vi "Write Configuration File.vi"() -> ()   [LabVIEW 2016]
uses:
  Hardware Configuration Controls/Company.ctl
  Hardware Configuration Controls/Device Type.ctl
  Hardware Configuration Controls/Device Function.ctl
panel:
  in  "Quit":bool
  in  "Save File":bool
  in  "Load File":bool
  in  "Configuration Name":string
  in  "Hardware Configuration Information":T4(array[cluster])
  # "Make sure the 0 element of the array is\nwhere you start putting port/id info"
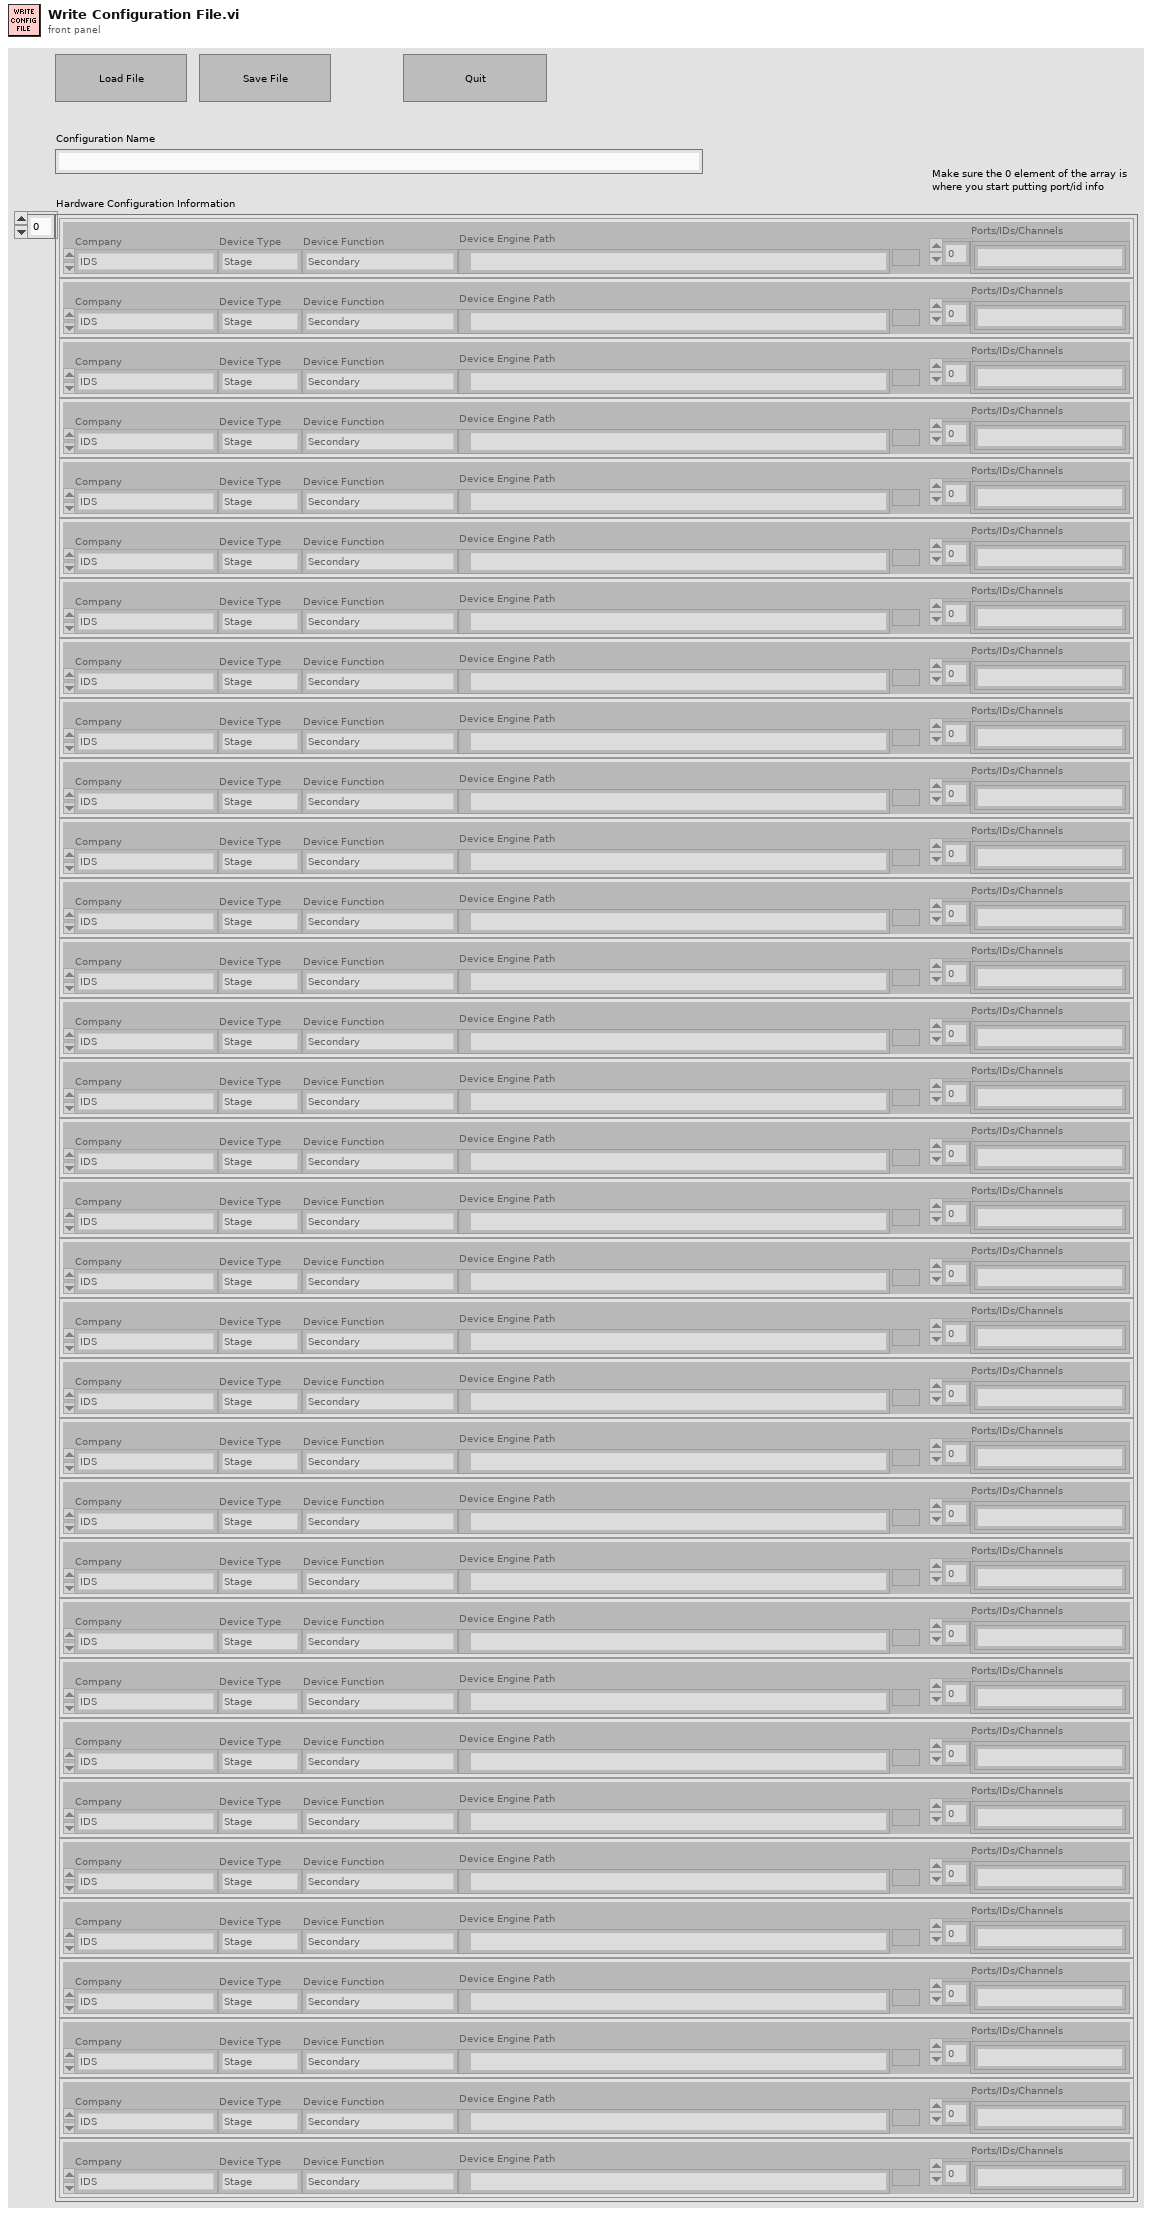
[diagram p1: front panel]
types:
  T1 = typedef "Company.ctl" = enum16{"ASI", "Coherent", "CVI", "Hamamatsu", "IDS", "Mad City Labs", "Marzhauser", "Measurement Computing", "MPB Com", "Photometrics", "PI", "Prior", "Thorlabs"}
  T2 = typedef "Device Type.ctl" = enum16{"AOTF", "Camera", "Deformable Mirror", "Laser", "Shutter", "Stage"}
  T3 = typedef "Device Function.ctl" = enum16{"Primary", "Secondary", "Overview", "Wide Field Drift Correction", "642 nm Excitation", "560 nm Excitation", "546 nm Excitation", "488 nm Excitation", "405 nm Excitation", "Objective Drift Correction", "Objective XY", "Objective Z", "Sample XY", "Sample Coarse Z", "Sample Z", "4Pi Lower", "4Pi Upper", "Adj Cavity"}
  T4 = cluster{"Company":T1, "Device Type":T2, "Device Function":T3, "Device Engine Path":path, "Ports/IDs/Channels":string[]}[]
  T5 = cluster{"Company":T1, "Device Type":T2, "Device Function":T3, path, "Device Port/ID/Channel Info":string[]}
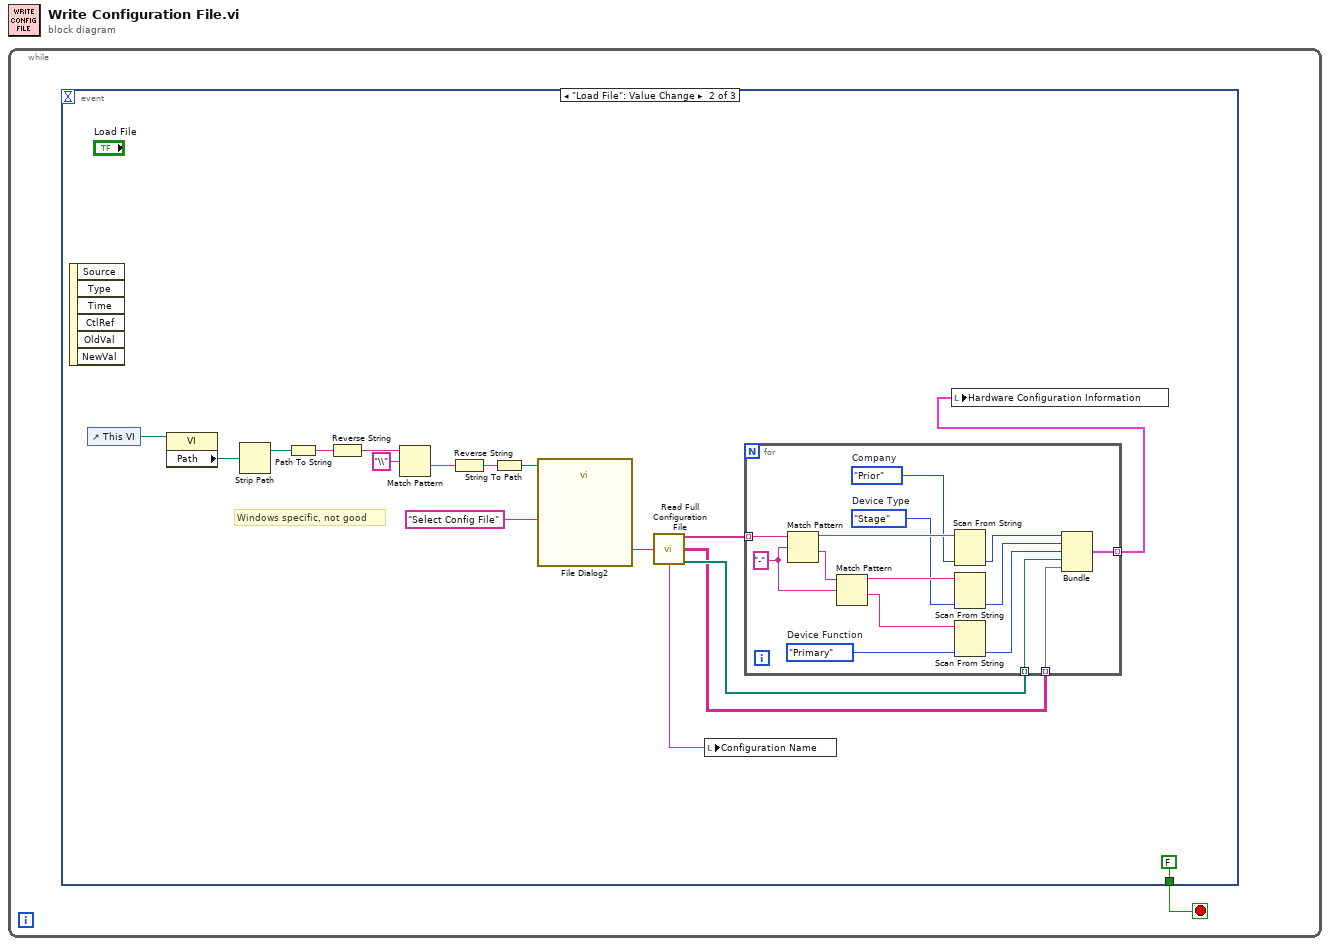
[diagram p0: block diagram]
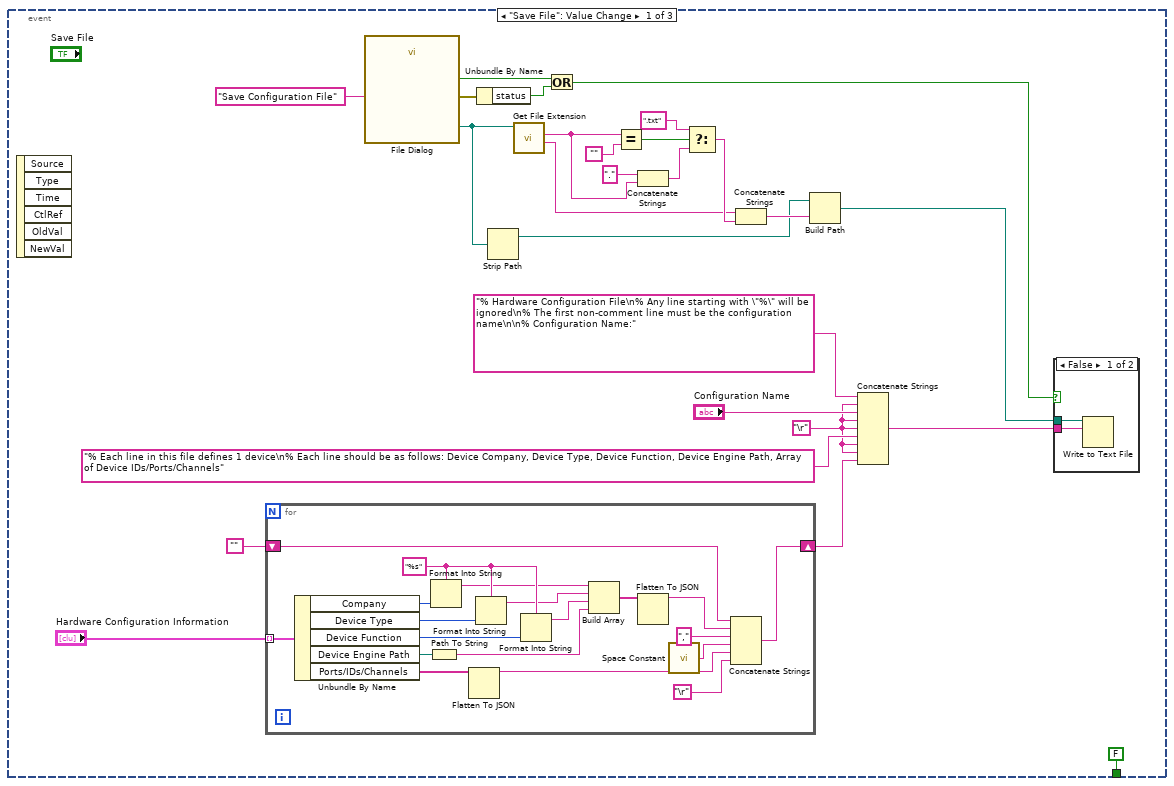
[diagram p2: hidden frame]
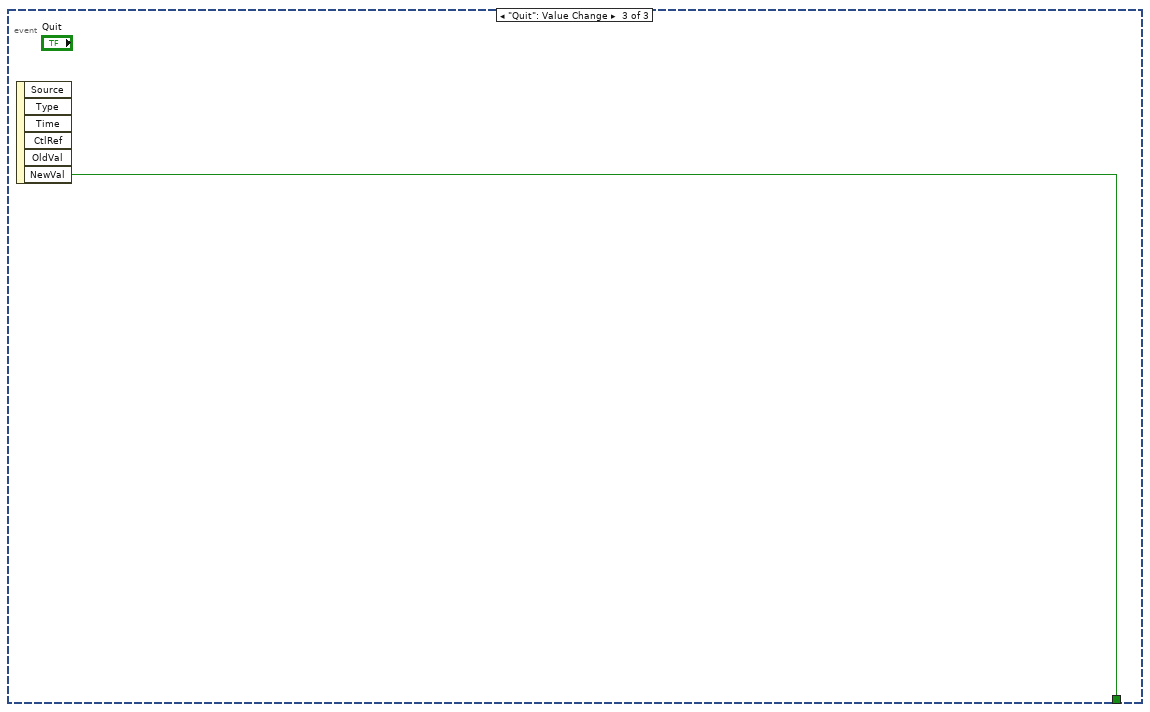
[diagram p4: hidden frame]
diagram:
  n1 = while {
    stop <- w1 stop-if-true
    n2 = event shown="[1] \"Load File\": Value Change" {
      selector: _ -> [_ _ _]
      dyn-events: _ -> [_ _ _]
      timeout: _ -> [_ _ _]
      tunnel: [FALSE ("NewVal") FALSE ("NewVal") w81] -> w1
      event "Save File": Value Change {
        w10 = "\r"
        n3 = event-data() -> ()  [unwired: 1 in, 6 out]
        n4 = for {
          tunnel: "Hardware Configuration Information" -> [w46] mode=indexing
          shift-right: [w30] -> w9
          shift-left: "" -> [w32]
          w44 = "%s" ("format string")
          n5 = Unbundle By Name(w46) -> ("Company"=w45:T1, "Device Type"=w43:T2, "Device Function"=w42:T3, "Device Engine Path"=w41:path, "Ports/IDs/Channels"=w35:string[])
          n6 = Path To String(path=w41) -> (string=w39:string)
          n7 = Format Into String(format string=w44, w45) -> (resulting string=w40:string)  [unwired: 2 in, 1 out]
          n8 = Flatten To JSON(anything=w35) -> (JSON string=w34:string)  [unwired: 2 in, 1 out]
          n9 = Format Into String(format string=w44, w43) -> (resulting string=w38:string)  [unwired: 2 in, 1 out]
          n10 = Format Into String(format string=w44, w42) -> (resulting string=w37:string)  [unwired: 2 in, 1 out]
          n11 = Build Array(w40, w38, w37, w39) -> (w36:string[])
          n12 = Flatten To JSON(anything=w36) -> (JSON string=w33:string)  [unwired: 2 in, 1 out]
          n13 = call <vilib>:"Space Constant.vi"() -> ("String"=w47:string)
          n14 = Concatenate Strings(w32, w33, ",", w47, w34, "\r") -> (w30:string)
        }
        n15 = call "File Dialog"("prompt"="Save Configuration File") -> ("selected path"=w6:path, "cancelled"=w25:bool, "error out"=w26:errorcluster)  [unwired: 11 in, 1 out]
        n16 = Unbundle By Name(w26) -> ("status"=w24:bool)
        n17 = Strip Path(path=w6) -> (stripped path=w5:path)  [unwired: 1 out]
        n18 = call <vilib>:"Get File Extension.vi"("file"=w6) -> ("filename without extension"=w19:string, "lowercase file extension"=w17:string)  [unwired: 6 in, 3 out]
        n19 = Or(x=w25, y=w24) -> (x .or. y?=w4:bool)
        n20 = Equal?(x=w17, y="") -> (x = y?=w23:bool)
        n21 = Concatenate Strings(".", w17) -> (w16:string)
        n22 = Select(t=".txt" ("prompt"), s=w23, f=w16) -> (s? t:f=w20:string)
        n23 = Concatenate Strings(w19, w20) -> (w7:string)
        n24 = Build Path(base path=w5, name or relative path=w7) -> (appended path=w3:path)
        n25 = Concatenate Strings("% Hardware Configuration File\n% Any line starting with \"%\" will be ignored\n% The first non-comment line must be the configuration name\n\n% Configuration Name:" ("format string"), w10, "Configuration Name", w10, w10, "% Each line in this file defines 1 device\n% Each line should be as follows: Device Company, Device Type, Device Function, Device Engine Path, Array of Device IDs/Ports/Channels" ("format string"), w10, w10, w9) -> (w8:string)
        n26 = case shown="False" w4 {
          tunnel: w8 -> [w29 _]
          tunnel: w3 -> [w28 _]
          frame False {
            n27 = Write to Text File(file (use dialog)=w28, text=w29) -> ()  [unwired: 2 in, 3 out]
          }
          frame True {
          }
        }
      }
      event "Load File": Value Change {
        # "Windows specific, not good"
        n28 = event-data() -> ()  [unwired: 1 in, 6 out]
        n29 = control-ref of="This VI"() -> (w64:refnum<vi>)
        n30 = property class="VI"(reference=w64) -> ("Path"=w63:path)  [unwired: 1 in, 2 out]
        n31 = Strip Path(path=w63) -> (stripped path=w62:path)  [unwired: 1 out]
        n32 = Path To String(path=w62) -> (string=w61:string)
        n33 = Reverse String(1:w61) -> (0:w60:string)
        n34 = Match Pattern(string=w60, regular expression="\\") -> (after substring=w58:string)  [unwired: 1 in, 3 out]
        n35 = Reverse String(1:w58) -> (0:w57:string)
        n36 = String To Path(string=w57) -> (path=w55:path)
        n37 = call "File Dialog2"("start path"=w55, "prompt"="Select Config File") -> ("selected path"=w54:path)  [unwired: 10 in, 3 out]
        n38 = call "Read Full Configuration File.vi"("Config File Path"=w54) -> ("Unique Notifier Names"=w52:string[], "Device Port/ID/Channel Info"=w50:string[][], "Configuration Name"=w53:string, "Device Engine Paths"=w51:path[])  [unwired: 11 in]
        n39 = local write "Configuration Name"(w53) -> ()
        n40 = for {
          tunnel: w52 -> [w80] mode=indexing
          tunnel: w51 -> [w77] mode=indexing
          tunnel: w50 -> [w76] mode=indexing
          tunnel: [w75] -> w49 mode=indexing
          w70 = Device_Function."Primary"  # Device Function
          w71 = Device_Type."Stage"  # Device Type
          w72 = Company."Prior"  # Company
          w78 = "-"
          n41 = Match Pattern(string=w80, regular expression=w78) -> (before substring=w74:string, after substring=w79:string)  [unwired: 1 in, 2 out]
          n42 = Match Pattern(string=w79, regular expression=w78) -> (before substring=w73:string, after substring=w66:string)  [unwired: 1 in, 2 out]
          n43 = Scan From String(input string=w74, default 1=w72) -> (output 1=w69:T1)  [unwired: 3 in, 3 out]
          n44 = Scan From String(input string=w73, default 1=w71) -> (output 1=w68:T2)  [unwired: 3 in, 3 out]
          n45 = Scan From String(input string=w66, default 1=w70) -> (output 1=w67:T3)  [unwired: 3 in, 3 out]
          n46 = Bundle("Company"=w69, "Device Type"=w68, "Device Function"=w67, w77, "Device Port/ID/Channel Info"=w76) -> (w75:T5)  [unwired: 1 in]
        }
        n47 = local write "Hardware Configuration Information"(w49) -> ()
      }
      event "Quit": Value Change {
        n48 = event-data() -> ("NewVal"=w81:bool)  [unwired: 1 in, 5 out]
      }
    }
  }
